vi "VariaveisTaskMedicao.vi"() -> ()   [LabVIEW 2019]
panel:
  out "Medicoes":bool
  in  "Anemômetro2":dbl
  in  "Anemômetro1":dbl
  in  "CorrenteAeroGerador":dbl
  in  "TensaoAeroGerador":dbl
  out "AnalogTasks":cluster{"Function":i32, "Task":refnum<k21>}[](array[cluster])
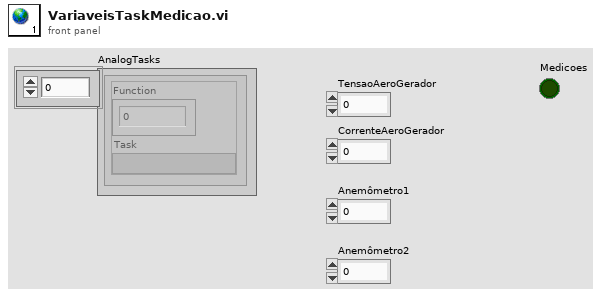
[diagram p1: front panel]
diagram:
